vi "4110_Create V Chans.vi"(5 "Device Ref in":T1 format="%.0x", 7 "# of V Channels to Add?":i16, 8 "error in":errorcluster, 9 "sense":T2=1008 caption="sense (out)" items=["Local"=1008, "Remote"=1009], 10 "Current Limit":dbl, 11 "Init Value":dbl) -> (0 "error out":errorcluster)   [LabVIEW 2018]
uses:
  <vilib>/NI VeriStand/Custom Device API/Custom Device API.lvlib
  <vilib>/NI Veristand/Custom Device API/Set Item Property (U16).vi
  <vilib>/NI Veristand/Custom Device API/Custom Device Channel Type.ctl
  <vilib>/NI Veristand/Custom Device API/Custom Device Channel.ctl
  <vilib>/NI Veristand/Custom Device API/Get Item Property (U16).vi
  4110_Global.vi
  NI PXI-4110 Programmable Power Supply Custom Device.lvlib
  <instrlib>/niDCPower/nidcpower.llb/niDCPower Sense.ctl
  <vilib>/NI Veristand/Custom Device API/Custom Device Item Ref.ctl
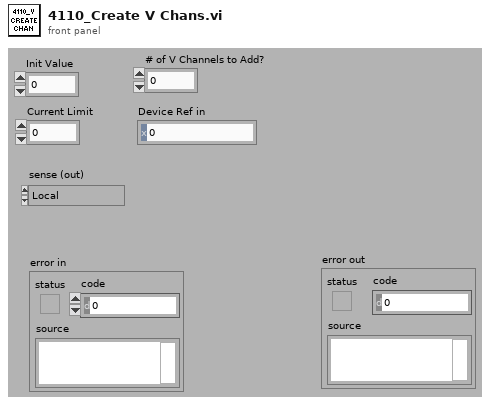
[diagram p1: front panel]
types:
  T1 = typedef "Custom Device API.lvlib/Custom Device Item Ref.ctl" = u64
  T2 = typedef "niDCPower Sense.ctl" = i32
  T3 = typedef "Custom Device API.lvlib/Custom Device Channel.ctl" = cluster{"Type":T4, "Units":string, "Default Value":dbl, "Faultable":bool, "Scalable":bool}
  T4 = typedef "Custom Device API.lvlib/Custom Device Channel Type.ctl" = enum16{"Input", "Output"}
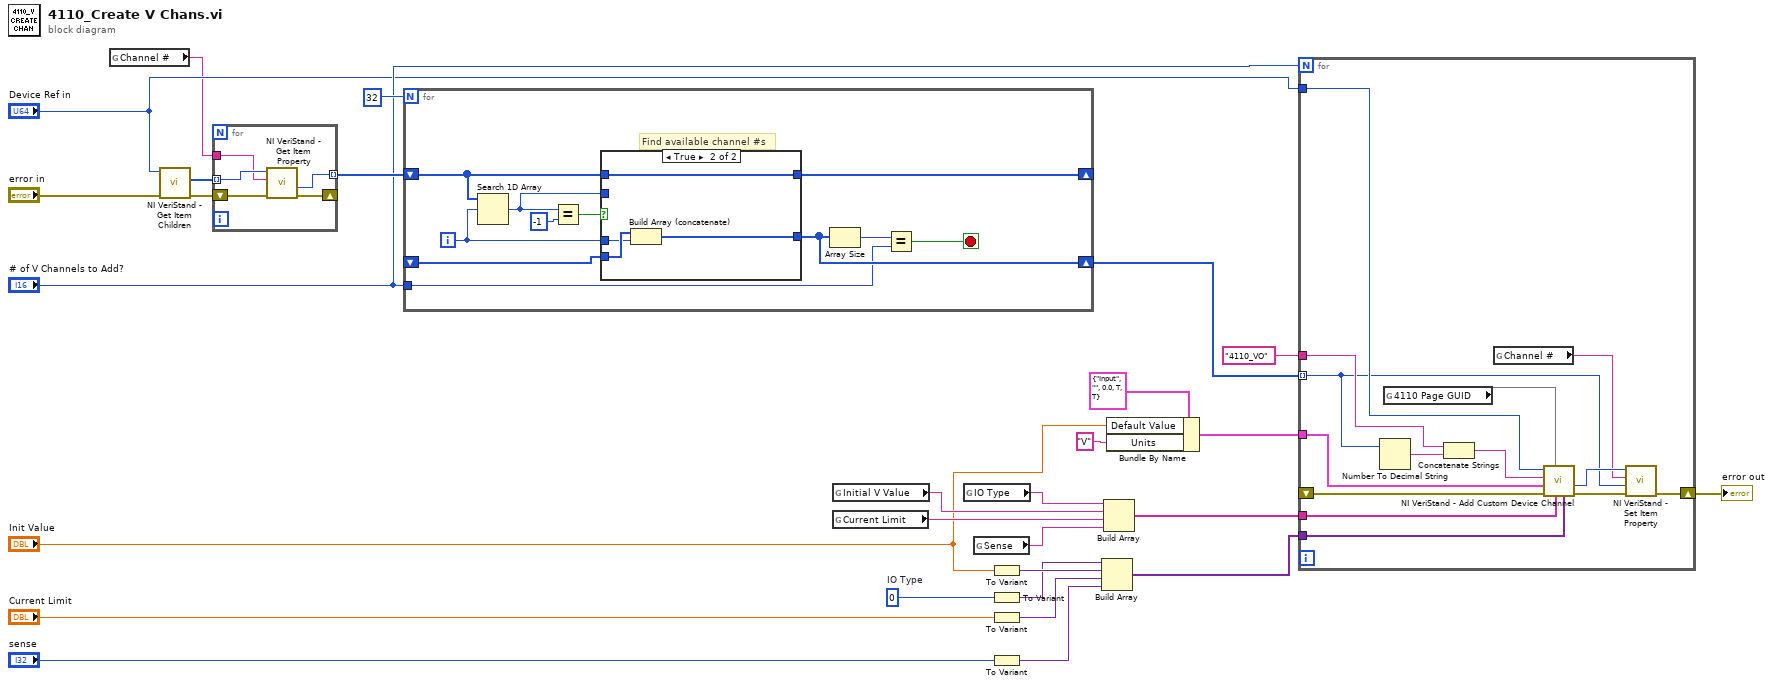
[diagram p0: block diagram]
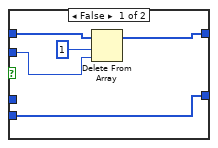
[diagram p2: hidden frame]
diagram:
  w5 = u16 0  # IO Type
  n1 = global read "4110_Global.vi" "Channel #"() -> (w10:string)
  n2 = call <vilib>:"NI VeriStand - Get Item Children.vi"("error in (no error)"="error in", "Item Ref in"="Device Ref in") -> ("error out"=w18:errorcluster, "Child Refs"=w19:T1[])  [unwired: 6 in, 2 out]
  n3 = for {
    tunnel: w19 -> [w33] mode=indexing
    shift-right: [w30] -> _
    shift-left: w18 -> [w32]
    tunnel: w10 -> [w31]
    tunnel: [w29] -> w17 mode=indexing
    n4 = call-poly <vilib>:"NI VeriStand - Get Item Property.vi"("error in (no error)"=w32, "Property Name"=w31, "Item Ref in"=w33) -> ("error out"=w30:errorcluster, "Value"=w29:u16)  [unwired: 5 in, 2 out]
  }
  n5 = for {
    N: 32 -> [_]
    shift-right: [w37] -> w16
    shift-left: _ -> [w42]
    shift-right: [w38] -> _
    shift-left: w17 -> [w40]
    tunnel: "# of V Channels to Add?" -> [w35]
    i -> [w41]
    stop <- w34 stop-if-true
    # "Find available channel #s"
    n6 = Search 1D Array(1D array=w40, element=w41) -> (index of element=w39:i32)  [unwired: 1 in]
    n7 = Equal?(x=w39, y=-1) -> (x = y?=w43:bool)
    n8 = case shown="True" w43 {
      tunnel: w42 -> [w49 w53]
      tunnel: [w49 w52] -> w37
      tunnel: w41 -> [_ w51]
      tunnel: w40 -> [w48 w50]
      tunnel: w39 -> [w46 _]
      tunnel: [w45 w50] -> w38
      frame False {
        n9 = Delete From Array(array=w48, length=1, index=w46) -> (array with subset deleted=w45:u16[])  [unwired: 1 out]
      }
      frame True {
        n10 = Build Array (concatenate)(w53, w51) -> (w52:i32[])
      }
    }
    n11 = Array Size(array=w37) -> (size(s)=w36:i32)
    n12 = Equal?(x=w36, y=w35) -> (x = y?=w34:bool)
  }
  n13 = global read "4110_Global.vi" "Initial V Value"() -> (w8:string)
  n14 = global read "4110_Global.vi" "Current Limit"() -> (w7:string)
  n15 = global read "4110_Global.vi" "IO Type"() -> (w9:string)
  n16 = global read "4110_Global.vi" "Sense"() -> (w6:string)
  n17 = To Variant(anything="Init Value") -> (Variant=w24:variant)
  n18 = To Variant(anything=w5) -> (Variant=w23:variant)
  n19 = To Variant(anything="Current Limit") -> (Variant=w25:variant)
  n20 = To Variant(anything="sense") -> (Variant=w26:variant)
  n21 = Build Array(w23, w24, w25, w26) -> (w27:variant[])
  n22 = Build Array(w9, w8, w7, w6) -> (w28:string[])
  n23 = Bundle By Name(cluster=T3 {"Type"=enum."Input", "Units"="", "Default Value"=0.0, "Faultable"=TRUE, "Scalable"=TRUE} ("Channel"), "Default Value"="Init Value", "Units"="V") -> (w14:T3)
  n24 = for {
    N: "# of V Channels to Add?" -> [_]
    shift-right: [w60] -> w21
    shift-left: _ -> [w67]
    tunnel: w14 -> [w66]
    tunnel: "Device Ref in" -> [w65]
    tunnel: "4110_VO" -> [w64]
    tunnel: w27 -> [w58]
    tunnel: w28 -> [w57]
    tunnel: w16 -> [w56] mode=indexing
    n25 = Number To Decimal String(number=w56) -> (decimal integer string=w63:string)  [unwired: 1 in]
    n26 = global read "4110_Global.vi" "4110 Page GUID"() -> (w54)
    n27 = Concatenate Strings(w64, w63) -> (w62:string)
    n28 = global read "4110_Global.vi" "Channel #"() -> (w55:string)
    n29 = call <vilib>:"NI VeriStand - Add Custom Device Channel.vi"("Property Values"=w58, "Property names"=w57, "GUID (Default Channel)"=w54, "error in (no error)"=w67, "Channel"=w66, "Channel Name"=w62, "Parent Ref in"=w65) -> ("error out"=w61:errorcluster, "Channel Ref"=w59:T1)  [unwired: 1 in, 2 out]
    n30 = call-poly <vilib>:"NI VeriStand - Set Item Property.vi"("error in (no error)"=w61, "Value"=w56, "Property Name"=w55, "Item Ref in"=w59) -> ("error out"=w60:errorcluster)  [unwired: 5 in, 2 out]
  }
  "error out" <- w21
